vi "Get Pattern.vi"(11 "Switch File Interface in":refnum<class "Switch File Interface.lvclass">) -> (2 "file extension":string)   [LabVIEW 2018, in "Switch System Explorer.lvlib" / "Switch File Interface.lvclass"]
uses:
  Switch Configuration.llb/Switch File Interface.lvclass
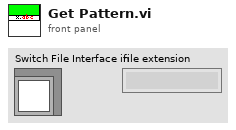
[diagram p1: front panel]
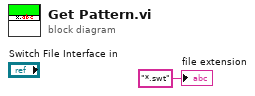
[diagram p0: block diagram]
diagram:
  "file extension" <- "*.swt" ("file extension")
